vi "2D_array_zu_punktspur.vi"(7 "Color":u32, 8 "größe":sgl, 9 "Array":dbl[][](array[numeric]), 10 "dimension size":i32, 11 "Refnum in":T1) -> (3 "Refnum out":T1)   [LabVIEW 2014]
uses:
  <vilib>/vision/Image Controls.llb/IMAQ Image.ctl
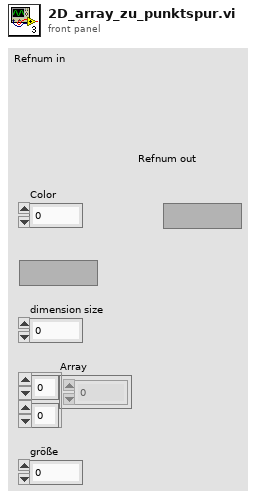
[diagram p1: front panel]
types:
  T1 = typedef "IMAQ Image.ctl" = refnum<image>
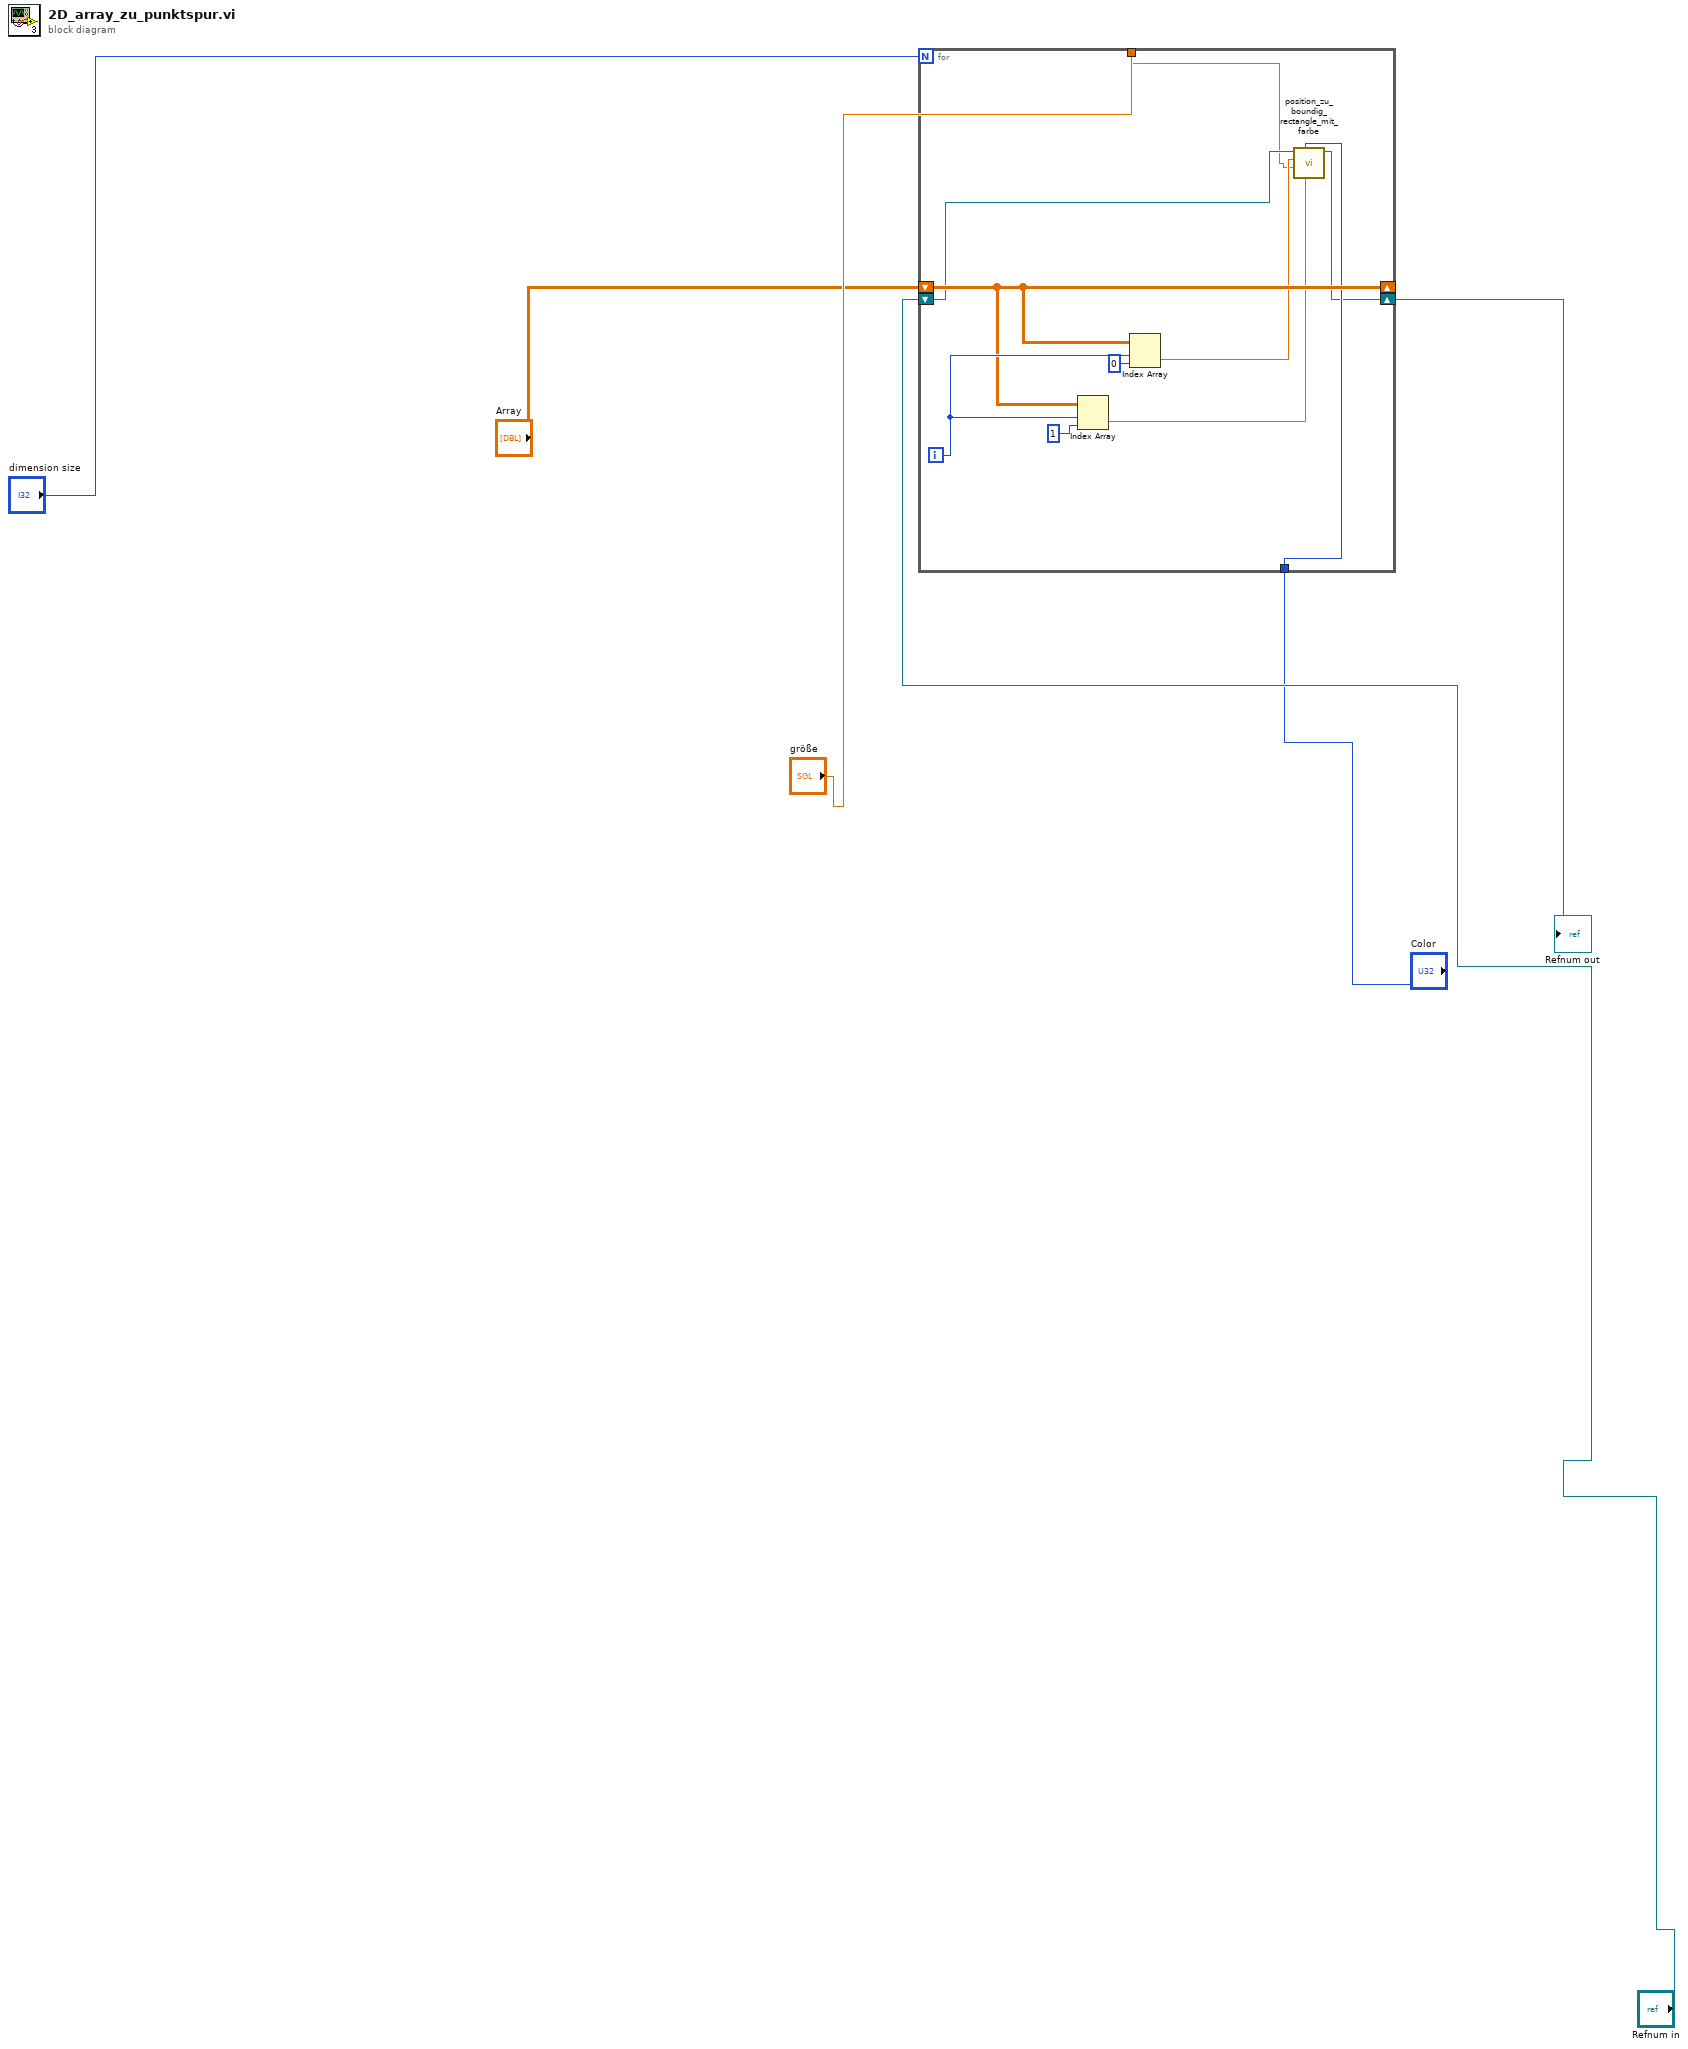
[diagram p0: block diagram]
diagram:
  n1 = for {
    N: "dimension size" -> [_]
    shift-right: [w10] -> w2
    shift-left: "Refnum in" -> [w11]
    shift-right: [w13] -> _
    shift-left: "Array" -> [w13]
    tunnel: "größe" -> [w7]
    tunnel: "Color" -> [w12]
    i -> [w15]
    n2 = Index Array(array=w13, index (row)=w15, index (col)=1 ("disabled index (col)")) -> (element=w8:dbl)
    n3 = Index Array(array=w13, index (row)=w15, index (col)=0) -> (element=w9:dbl)
    n4 = call "position_zu_boundig_rectangle_mit_farbe.vi"("y"=w8, "Color"=w12, "größe in"=w7, "x"=w9, "Refnum in"=w11) -> ("Refnum out"=w10:T1)  [unwired: 6 in]
  }
  "Refnum out" <- w2
